vi "controlpanel.vi"() -> ()   [LabVIEW 2018]
uses:
  <vilib>/Platform/TimedLoop/XDataNode/timing_clust.ctl
  <vilib>/Platform/TimedLoop/XDataNode/nitl_modes.ctl
  <vilib>/Platform/TimedLoop/XDataNode/wakeup.ctl
  <vilib>/platform/TimedLoop/XDataNode/XDataNode.xnode
  <vilib>/Platform/TimedLoop/XDataNode/XDNodeRunTimeDep.lvlib
panel:
  out "Output":bool[](array[boolean])
  in  "Input":bool[](array[boolean])
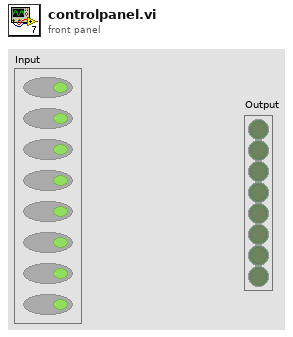
[diagram p1: front panel]
types:
  T1 = typedef "XDNodeRunTimeDep.lvlib/timing_clust.ctl" = cluster{"Expected End [f-1]":u64, "Actual End [f-1]":u64, "Finished Late? [f-1]":bool, "Expected End [i-1]":u64, "Actual End [i-1]":u64, "Finished Late? [i-1]":bool, "Expected Start [i]":u64, "Actual Start [i]":u64, "Expected Start [f]":u64, "Actual Start [f]":u64, "Source Name":string, "Structure Name":string, "Period":i64, "Deadline":i64, "Offset":i64, "Start":i64, "Priority":i32, "Timeout":i32, "Mode":T2, "Wakeup Reason":T3, "Error":errorcluster, "Source Type":string, "Secondary Source Type":string, "Global End Time":u64, "Global Start Time":u64, "Frame Duration":u64, "Iteration Duration":u64, "Assigned CPU":i32, "I/O Scan Engine Mode":u32}
  T2 = typedef "XDNodeRunTimeDep.lvlib/nitl_modes.ctl" = enum32{"No Change", "Process missed periods, maintain original phase", "Discard missed periods, maintain original phase", "Process missed periods, ignore original phase", "Discard missed periods, ignore original phase"}
  T3 = typedef "XDNodeRunTimeDep.lvlib/wakeup.ctl" = enum32{"Normal", "Aborted", "Asynchronous wakeup", "Timing source error", "Timed loop error", "Timeout"}
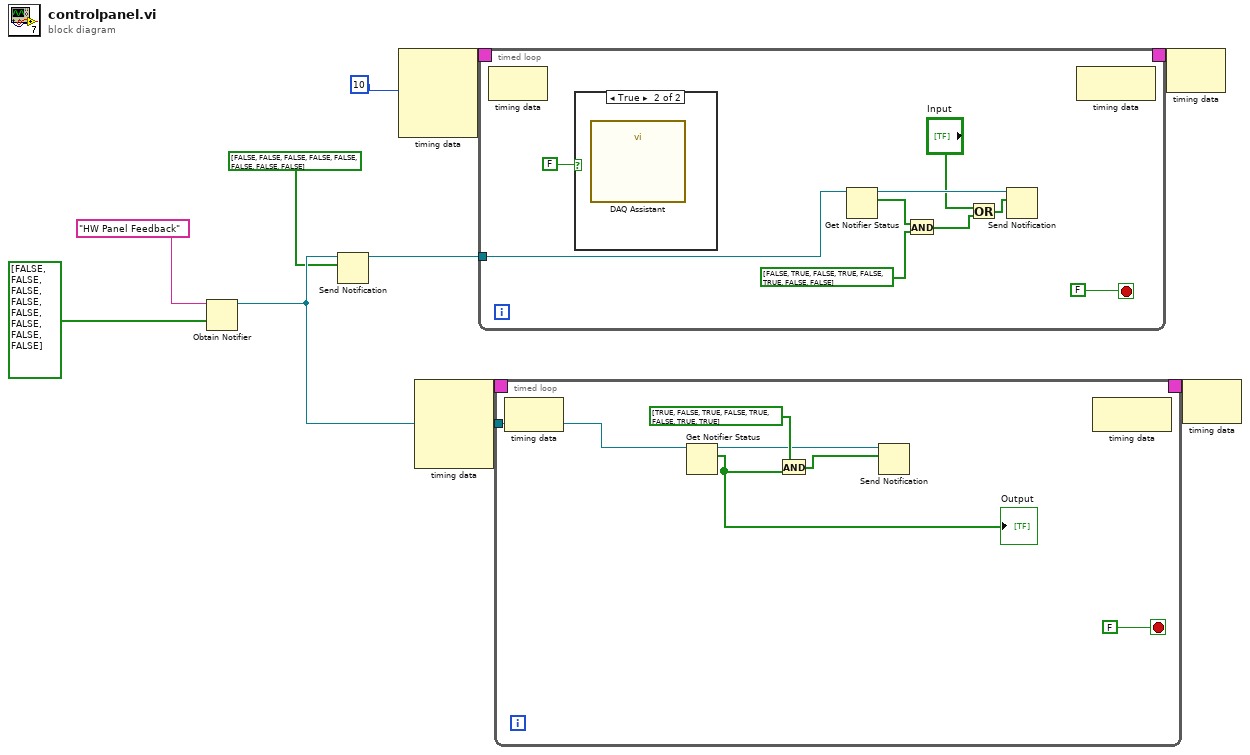
[diagram p0: block diagram]
diagram:
  n1 = Obtain Notifier(name (unnamed)="HW Panel Feedback", notification data type=bool[] [FALSE, FALSE, FALSE, FALSE, FALSE, FALSE, FALSE, FALSE]) -> (notifier out=w5:refnum<notifier>)  [unwired: 2 in, 2 out]
  n2 = Send Notification(notification=bool[] [FALSE, FALSE, FALSE, FALSE, FALSE, FALSE, FALSE, FALSE], notifier=w5) -> (notifier out=w4:refnum<notifier>)  [unwired: 1 in, 1 out]
  n3 = node-c288(10) -> (w10:T1)  [unwired: 3 in]
  n4 = node-c288() -> (w2:T1)  [unwired: 4 in]
  n5 = timed-loop {
    timing: w10 -> [_]
    timing-out: [_] -> w9
    tunnel: w4 -> [w17]
    stop <- FALSE stop-if-true
    n6 = node-c288() -> ()  [unwired: 1 in, 1 out]
    n7 = case shown="True" FALSE {
      frame False {
      }
      frame True {
        n8 = call "DAQ Assistant"() -> ()  [unwired: 17 in, 3 out]
      }
    }
    n9 = Get Notifier Status(notifier=w17) -> (notifier out=w16:refnum<notifier>, current notification=w15:bool[])  [unwired: 1 in, 3 out]
    n10 = And(x=w15, y=bool[] [FALSE, TRUE, FALSE, TRUE, FALSE, TRUE, FALSE, FALSE]) -> (x .and. y?=w11:bool[])
    n11 = Or(x="Input", y=w11) -> (x .or. y?=w13:bool[])
    n12 = Send Notification(notification=w13, notifier=w16) -> ()  [unwired: 1 in, 2 out]
    n13 = node-c288() -> ()  [unwired: 1 in, 1 out]
  }
  n14 = timed-loop {
    tunnel: w5 -> [w26]
    timing: w2 -> [_]
    timing-out: [_] -> w1
    stop <- FALSE stop-if-true
    n15 = node-c288() -> ()  [unwired: 1 in, 1 out]
    n16 = Get Notifier Status(notifier=w26) -> (notifier out=w24:refnum<notifier>, current notification=w22:bool[])  [unwired: 1 in, 3 out]
    "Output" <- w22
    n17 = And(x=bool[] [TRUE, FALSE, TRUE, FALSE, TRUE, FALSE, TRUE, TRUE], y=w22) -> (x .and. y?=w23:bool[])
    n18 = Send Notification(notification=w23, notifier=w24) -> ()  [unwired: 1 in, 2 out]
    n19 = node-c288() -> ()  [unwired: 1 in, 1 out]
  }
  n20 = node-c288(w9) -> ()  [unwired: 1 out]
  n21 = node-c288(w1) -> ()  [unwired: 1 out]
